vi "Unflatten.vi"(0 "Subroutine in":refnum<class "Subroutine.lvclass">, 1 "Linked List Ref":refnum<data-value>, 5 "Flattened Test Executive":string, 9 "Linked List ID":string, 11 "error in (no error)":errorcluster, 12 "Persistence in":refnum<class "IPersist.lvclass">, 13 "Compatibility Helper":refnum<class "ICompatibility Helper.lvclass">, 14 "Path Builder":refnum<class "IPath Builder.lvclass">) -> (3 "Linked List Ref out":refnum<data-value>, 6 "Flattened Test Executive out":string, 15 "error out":errorcluster)   [LabVIEW 2017, in "Test Executive.lvlib" / "Subroutine.lvclass"]
uses:
  <vilib>/gpm_packages/@cs/test-executive/Source/Test Executive/Subroutine/Subroutine.lvclass
  <vilib>/gpm_packages/@cs/persistence/source/IPersist/IPersist.lvclass
  <vilib>/gpm_packages/@cs/linked-list/Source/Linked List/ILinkedList/ILinked List.lvclass
  <vilib>/gpm_packages/@cs/test-executive/Source/Path Builder/IPath Builder/IPath Builder.lvclass
  <vilib>/gpm_packages/@cs/test-executive/Source/Compatibility Helper/ICompatibility Helper.lvclass
  <vilib>/gpm_packages/@cs/test-executive/Source/Test Executive/Executioner/Executioner.lvclass
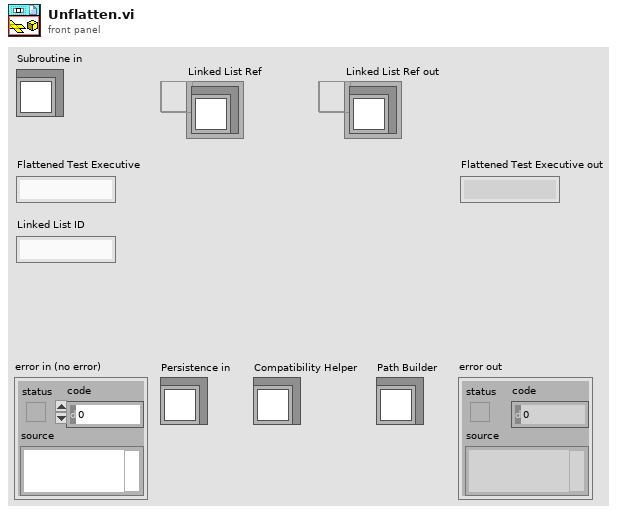
[diagram p1: front panel]
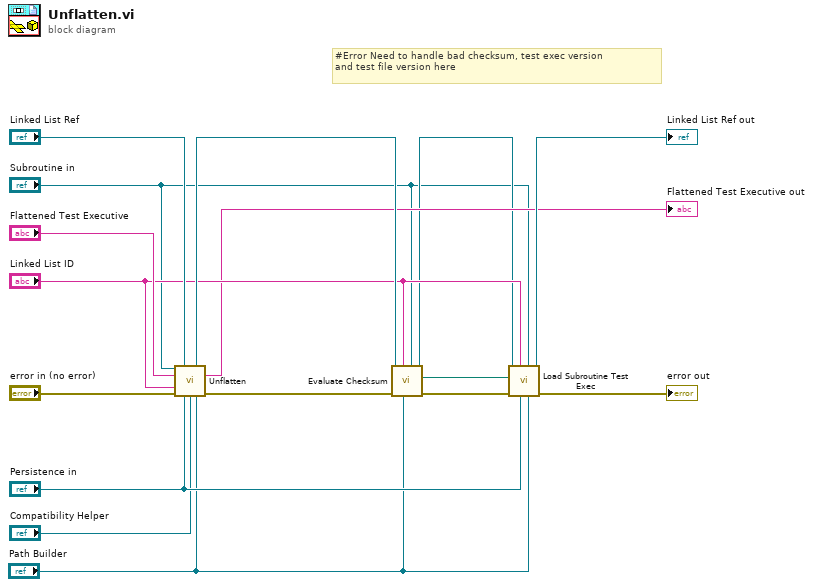
[diagram p0: block diagram]
diagram:
  # "#Error Need to handle bad checksum, test exec version\nand test file version here"
  n1 = call-parent "Unflatten.vi"("Executioner in"="Subroutine in", "Linked List Ref"="Linked List Ref", "Flattened Test Executive"="Flattened Test Executive", "Linked List ID"="Linked List ID", "error in (no error)"="error in (no error)", "Persistence in"="Persistence in", "Compatibility Helper"="Compatibility Helper", "Path Builder"="Path Builder") -> ("Linked List Ref out"=w9:refnum<data-value>, "Flattened Test Executive out"=→"Flattened Test Executive out":string, "error out"=w11:errorcluster)  [unwired: 5 in]
  n2 = call <vilib>:"Evaluate Checksum.vi"("Subroutine in"="Subroutine in", "Path Builder"="Path Builder", "Linked List ID"="Linked List ID", "error in (no error)"=w11, "Linked List Ref"=w9) -> ("error out"=w4:errorcluster, "Path"=w2:path, "Linked List Ref out"=w3:refnum<data-value>)  [unwired: 3 in, 1 out]
  n3 = call-dynamic "Load Subroutine Test Exec.vi"("Path Builder"="Path Builder", "Subroutine in"="Subroutine in", "Persistence in"="Persistence in", "Linked List ID"="Linked List ID", "error in (no error)"=w4, "Subroutine Path"=w2, "Linked List Ref"=w3) -> ("error out"=→"error out":errorcluster, "Linked List Ref out"=→"Linked List Ref out":refnum<data-value>)  [unwired: 1 in, 2 out]
